vi "同步D触发器（锁存）.vi"(1 "CP":bool, 3 "D":bool) -> (0 "Q":bool)   [LabVIEW 2012, in "触发器.lvlib"]
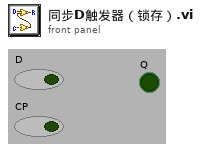
[diagram p1: front panel]
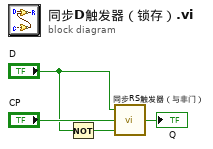
[diagram p0: block diagram]
diagram:
  n1 = Not(x="D") -> (.not. x?=w1:bool)
  n2 = call "同步RS触发器（与非门）.vi"("R"=w1, "CP"="CP", "S"="D") -> ("Q"=→"Q":bool)
